vi "FindStuff.vi"() -> ()   [LabVIEW 2014]
panel:
  out "Array":path[](array[path])
  in  "search pattern":string="*profile*"
  in  "Folders to Exclude":string[](array[string])=["Raw_Measurements", "Commands", "Results_Post_Processed", "Raw_Data", "Preferences", "Save_Plot", "Calibrations", "Raw_Calibrations", "gnuplots", "BL_plot", "File_Edits"]
  in  "File Path Control":path=path "/CentralDataCache"
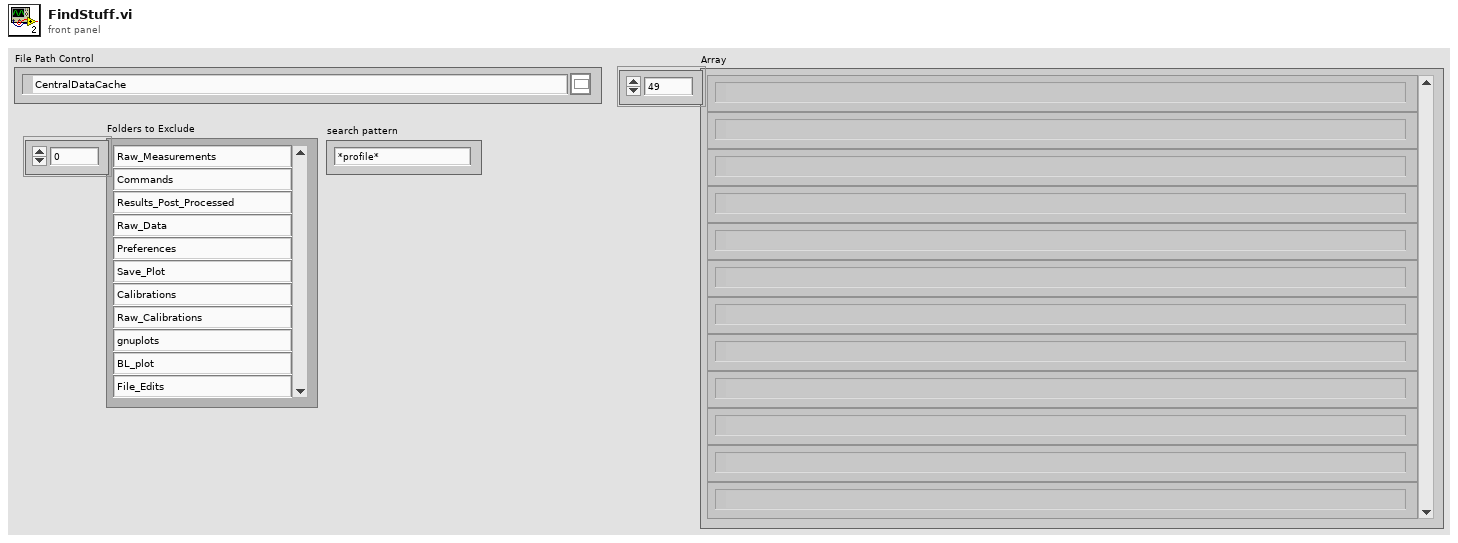
[diagram p1: front panel]
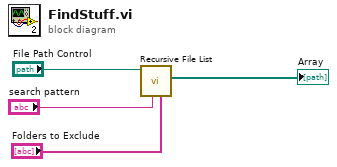
[diagram p0: block diagram]
diagram:
  n1 = call <vilib>:"Recursive File List.vi"("Folders to Exclude"="Folders to Exclude", "pattern"="search pattern", "Folder Path"="File Path Control") -> ("All Files in Dir"=→"Array":path[])  [unwired: 4 in, 4 out]
